vi "Data Ref FGV.vi"(5 "FIFO Idx Qs":T1, 7 "Command":T2=enum."Get", 8 "error in (no error)":errorcluster, 9 "From HWOutput Length":i32, 10 "To HWOutput Length":i32, 11 "From HWInput Length":i32) -> (0 "error out":errorcluster, 1 "From HWOutput FIFO Index / Length":i32, 2 "To HWOutput FIFO Index / Length":i32, 3 "From HWInput FIFO Index / Length":i32)   [LabVIEW 2016, in "Ballard Arinc-429 Engine.lvlib"]
uses:
  Ballard Arinc-429 Engine.lvlib
  RT Controls/Data Ref FGV Command.ctl
  RT Controls/FIFO Idx Qs.ctl
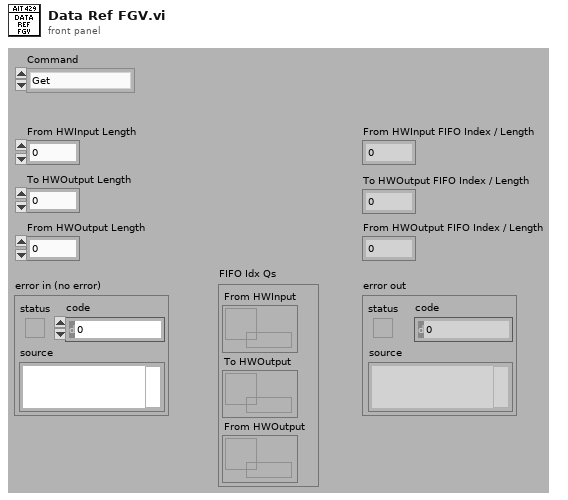
[diagram p1: front panel]
types:
  T1 = typedef "Ballard Arinc-429 Engine.lvlib/FIFO Idx Qs.ctl" = cluster{"From HWInput":refnum<queue>, "To HWOutput":refnum<queue>, "From HWOutput":refnum<queue>}
  T2 = typedef "Ballard Arinc-429 Engine.lvlib/Data Ref FGV Command.ctl" = enum16{"Intialize", "Get", "Update"}
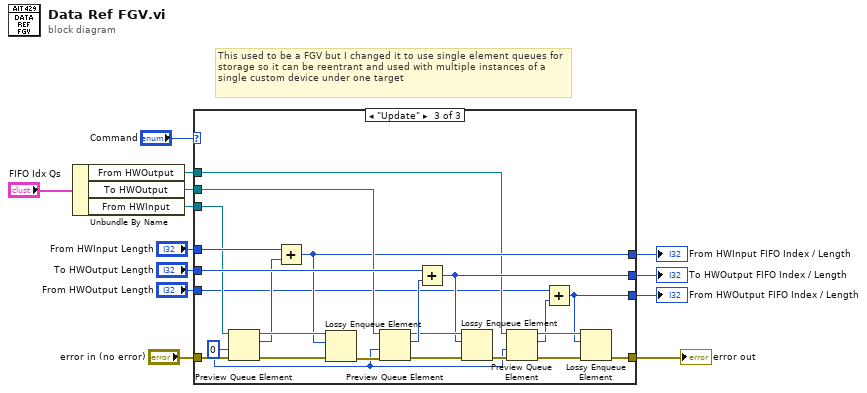
[diagram p0: block diagram]
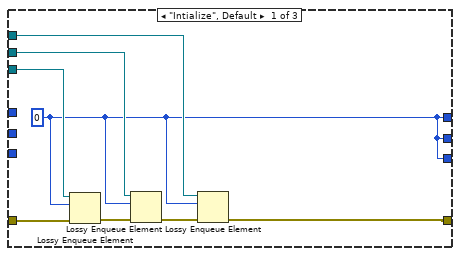
[diagram p2: hidden frame]
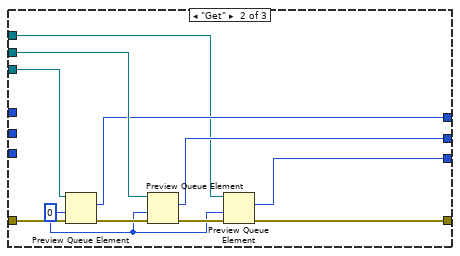
[diagram p3: hidden frame]
diagram:
  # "This used to be a FGV but I changed it to use single element queues for storage so it can be reentrant and used with multiple instances of a single custom device under one target"
  n1 = Unbundle By Name("FIFO Idx Qs") -> ("From HWOutput"=w1:refnum<queue>, "To HWOutput"=w5:refnum<queue>, "From HWInput"=w4:refnum<queue>)
  n2 = case shown="\"Update\"" "Command" {
    tunnel: "From HWInput Length" -> [_ _ w55]
    tunnel: "To HWOutput Length" -> [_ _ w54]
    tunnel: [w15 w28 w47] -> w10
    tunnel: [w15 w27 w44] -> w9
    tunnel: "error in (no error)" -> [w21 w32 w53]
    tunnel: [w14 w23 w37] -> w7
    tunnel: w4 -> [w19 w30 w52]
    tunnel: w5 -> [w18 w29 w51]
    tunnel: "From HWOutput Length" -> [_ _ w35]
    tunnel: [w15 w22 w34] -> w3
    tunnel: w1 -> [w16 w25 w36]
    frame "Intialize", Default {
      w15 = 0 ("index")
      n3 = Lossy Enqueue Element(queue=w19, element=w15, error in (no error)=w21) -> (error out=w20:errorcluster)  [unwired: 3 out]
      n4 = Lossy Enqueue Element(queue=w18, element=w15, error in (no error)=w20) -> (error out=w17:errorcluster)  [unwired: 3 out]
      n5 = Lossy Enqueue Element(queue=w16, element=w15, error in (no error)=w17) -> (error out=w14:errorcluster)  [unwired: 3 out]
    }
    frame "Get" {
      w24 = 0 ("timeout in ms (-1)")
      n6 = Preview Queue Element(queue=w30, timeout in ms (-1)=w24, error in (no error)=w32) -> (element=w28:i32, error out=w31:errorcluster)  [unwired: 2 out]
      n7 = Preview Queue Element(queue=w29, timeout in ms (-1)=w24, error in (no error)=w31) -> (element=w27:i32, error out=w26:errorcluster)  [unwired: 2 out]
      n8 = Preview Queue Element(queue=w25, timeout in ms (-1)=w24, error in (no error)=w26) -> (element=w22:i32, error out=w23:errorcluster)  [unwired: 2 out]
    }
    frame "Update" {
      w33 = 0 ("timeout in ms (-1)")
      n9 = Preview Queue Element(queue=w52, timeout in ms (-1)=w33, error in (no error)=w53) -> (queue out=w49:refnum<queue>, element=w48:i32, error out=w50:errorcluster)  [unwired: 1 out]
      n10 = Add(x=w55, y=w48) -> (x+y=w47:i32)
      n11 = Lossy Enqueue Element(queue=w49, element=w47, error in (no error)=w50) -> (error out=w43:errorcluster)  [unwired: 3 out]
      n12 = Preview Queue Element(queue=w51, timeout in ms (-1)=w33, error in (no error)=w43) -> (queue out=w45:refnum<queue>, element=w46:i32, error out=w42:errorcluster)  [unwired: 1 out]
      n13 = Add(x=w54, y=w46) -> (x+y=w44:i32)
      n14 = Lossy Enqueue Element(queue=w45, element=w44, error in (no error)=w42) -> (error out=w38:errorcluster)  [unwired: 3 out]
      n15 = Preview Queue Element(queue=w36, timeout in ms (-1)=w33, error in (no error)=w38) -> (queue out=w40:refnum<queue>, element=w39:i32, error out=w41:errorcluster)  [unwired: 1 out]
      n16 = Add(x=w35, y=w39) -> (x+y=w34:i32)
      n17 = Lossy Enqueue Element(queue=w40, element=w34, error in (no error)=w41) -> (error out=w37:errorcluster)  [unwired: 3 out]
    }
  }
  "From HWInput FIFO Index / Length" <- w10
  "To HWOutput FIFO Index / Length" <- w9
  "error out" <- w7
  "From HWOutput FIFO Index / Length" <- w3
